vi "create_files.vi"(11 "project name":string) -> (1 "converter2":path, 2 "converter1":path, 3 "controller":path)   [LabVIEW 2019]
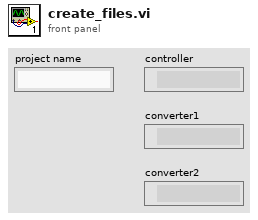
[diagram p1: front panel]
types:
  T1 = enum16{"open", "open or create", "create or replace", "create", "open (read only)"}
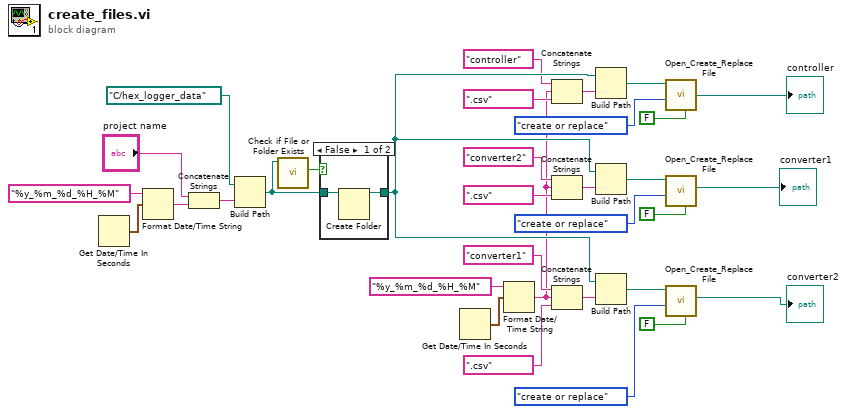
[diagram p0: block diagram]
diagram:
  n1 = Get Date/Time In Seconds() -> (seconds since 1Jan1904=w25:timestamp)
  n2 = Format Date/Time String(time format string (%c)="%y_%m_%d_%H_%M", seconds (now)=w25) -> (date/time string=w27:string)  [unwired: 1 in]
  n3 = Concatenate Strings("project name", w27) -> (w28:string)
  n4 = Build Path(base path=path "C:/hex_logger_data", name or relative path=w28) -> (appended path=w29:path)
  n5 = call <vilib>:"Check if File or Folder Exists.vi"("path"=w29) -> ("file or folder exists?"=w30:bool)  [unwired: 8 in, 2 out]
  n6 = case shown="False" w30 {
    tunnel: [w34 w36] -> w23
    tunnel: w29 -> [w35 w36]
    frame False {
      n7 = Create Folder(path (use dialog)=w35) -> (created path=w34:path)  [unwired: 2 in, 2 out]
    }
    frame True {
    }
  }
  n8 = Get Date/Time In Seconds() -> (seconds since 1Jan1904=w21:timestamp)
  n9 = Format Date/Time String(time format string (%c)="%y_%m_%d_%H_%M", seconds (now)=w21) -> (date/time string=w2:string)  [unwired: 1 in]
  n10 = Concatenate Strings("controller", w2, ".csv") -> (w14:string)
  n11 = Concatenate Strings("converter2", w2, ".csv") -> (w8:string)
  n12 = Concatenate Strings("converter1", w2, ".csv") -> (w20:string)
  n13 = Build Path(base path=w23, name or relative path=w14) -> (appended path=w11:path)
  n14 = Build Path(base path=w23, name or relative path=w8) -> (appended path=w5:path)
  n15 = Build Path(base path=w23, name or relative path=w20) -> (appended path=w17:path)
  n16 = call <vilib>:"Open_Create_Replace File.vi"("advisory dialog? (display:T)"=FALSE, "function (open:0)"=T1."create or replace", "file path"=w11) -> ("new file path"=→"controller":path)  [unwired: 5 in, 3 out]
  n17 = call <vilib>:"Open_Create_Replace File.vi"("advisory dialog? (display:T)"=FALSE, "function (open:0)"=T1."create or replace", "file path"=w5) -> ("new file path"=→"converter1":path)  [unwired: 5 in, 3 out]
  n18 = call <vilib>:"Open_Create_Replace File.vi"("advisory dialog? (display:T)"=FALSE, "function (open:0)"=T1."create or replace", "file path"=w17) -> ("new file path"=→"converter2":path)  [unwired: 5 in, 3 out]
